vi "subSwitches.vi"(1 "AxisId":i32=1, 2 "Index":i32=1) -> ()   [LabVIEW 2020]
panel:
  out "LimMaxSt":bool caption="S-MAX"
  out "LimMinSt":bool caption="S-MIN"
  in  "MaxPos":i32
  in  "MinPos":i32
  in  "LimMax":bool caption="S-MAX"
  in  "LimMin":bool caption="S-MIN"
  in  "REF4":bool caption="MAXSTP"
  in  "REF3":bool caption="MAXDEC"
  in  "REF2":bool caption="MINDEC"
  in  "REF1":bool caption="MINSTP"
  in  "RH4":bool caption="High"
  in  "RL4":bool caption="Low"
  in  "RH3":bool caption="High"
  in  "RL3":bool caption="Low"
  in  "RH2":bool caption="High"
  in  "RL2":bool caption="Low"
  in  "RH1":bool caption="High"
  in  "RL1":bool caption="Low"
  in  "MaxDec":bool caption="MAXDEC"
  in  "MinDec":bool caption="MINDEC"
  in  "MaxStop":bool caption="MAXSTOP"
  in  "MinStop":bool caption="MINSTOP"
  out "MaxDecSt":bool caption="MAXDEC"
  out "MinDecSt":bool caption="MINDEC"
  in  "Save":bool
  in  "H4":bool caption="High"
  in  "L4":bool caption="Low"
  in  "H3":bool caption="High"
  in  "L3":bool caption="Low"
  in  "H2":bool caption="High"
  in  "L2":bool caption="Low"
  in  "H1":bool caption="High"
  in  "L1":bool caption="Low"
  out "MaxStopSt":bool caption="MAXSTP"
  out "MinStopSt":bool caption="MINSTP"
  out "Hyst":i32 caption="Limit switch hysteresis"
  in  "Close":bool
  # "Axis"
  # "State (activated?)"
  # "Limit switches (mask + polarity)"
  # "Ref switch (mask + polarity)"
  # "Software limits"
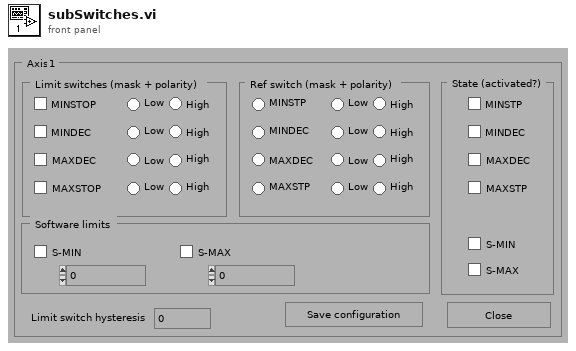
[diagram p1: front panel]
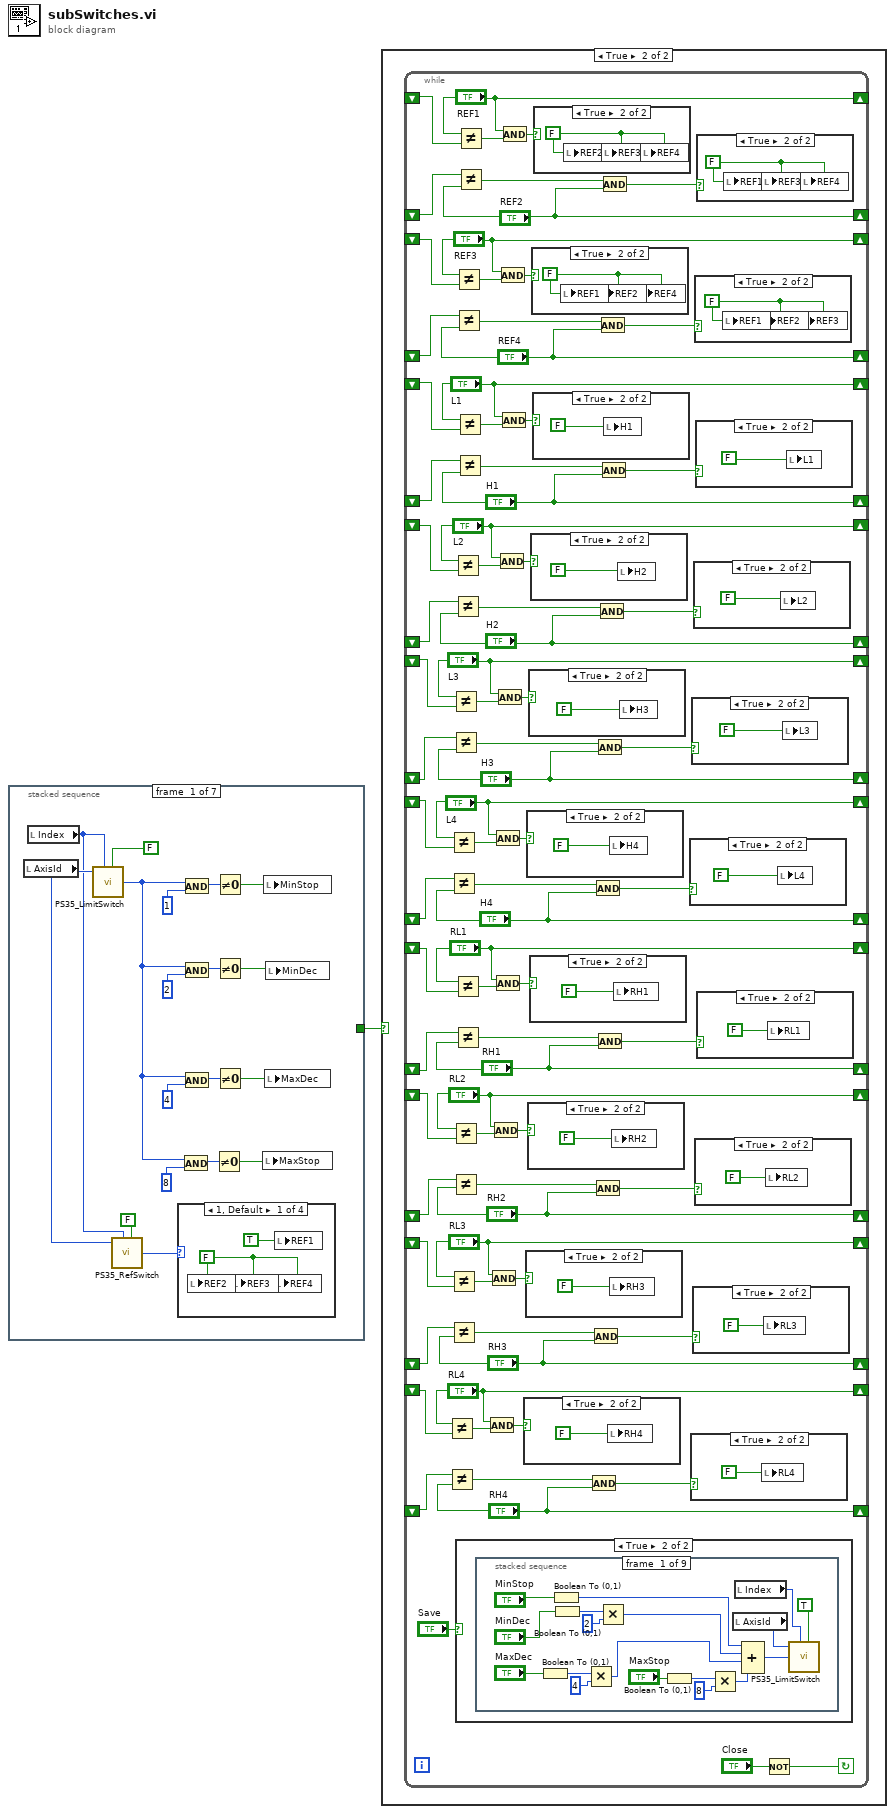
[diagram p0: block diagram]
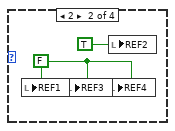
[diagram p2: hidden frame]
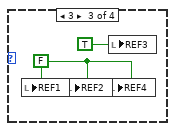
[diagram p3: hidden frame]
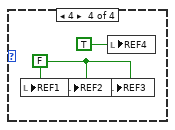
[diagram p4: hidden frame]
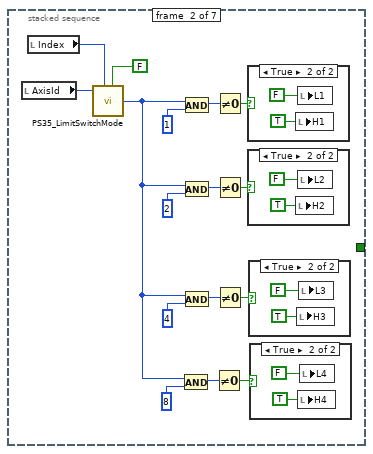
[diagram p5: hidden frame]
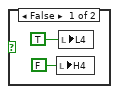
[diagram p6: hidden frame]
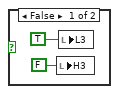
[diagram p7: hidden frame]
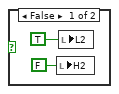
[diagram p8: hidden frame]
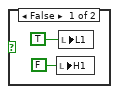
[diagram p9: hidden frame]
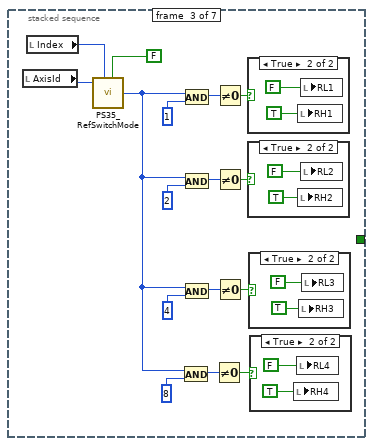
[diagram p10: hidden frame]
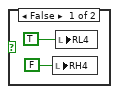
[diagram p11: hidden frame]
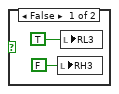
[diagram p12: hidden frame]
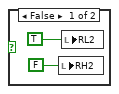
[diagram p13: hidden frame]
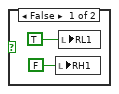
[diagram p14: hidden frame]
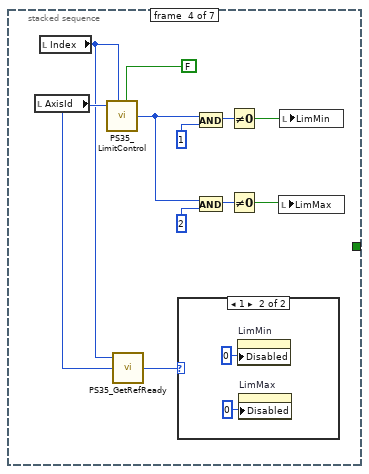
[diagram p15: hidden frame]
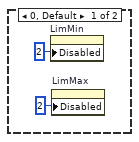
[diagram p16: hidden frame]
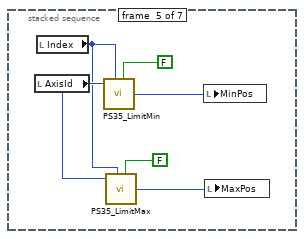
[diagram p17: hidden frame]
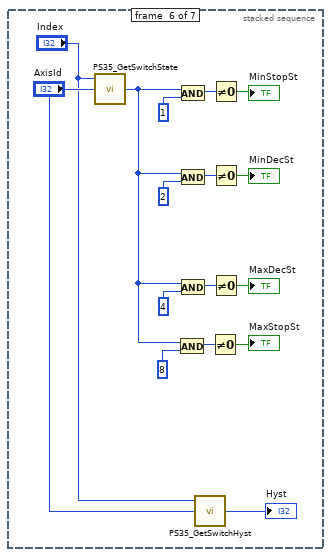
[diagram p18: hidden frame]
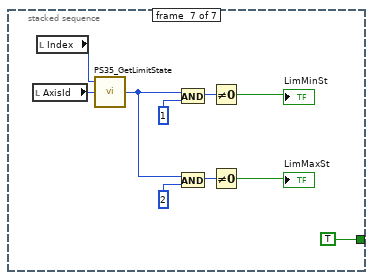
[diagram p19: hidden frame]
diagram:
  n1 = stacked-sequence {
    tunnel: [_ _ _ _ _ _ TRUE] -> w1
    frame #0 {
      n2 = local read "AxisId"() -> (w3:i32)
      n3 = local read "Index"() -> (w2:i32)
      n4 = call "PS35_LimitSwitch.vi"("Axis number"=w3, "Control unit ID"=w2, "function"=FALSE ("WriteRead")) -> ("Value-Out"=w10:i32)  [unwired: 5 in, 1 out]
      n5 = call "PS35_RefSwitch.vi"("Axis number"=w3, "Control unit ID"=w2, "function"=FALSE ("WriteRead")) -> ("Value-Out"=w4:i32)  [unwired: 5 in, 1 out]
      n6 = case shown="1, Default" w4 {
        frame 1, Default {
          w20 = FALSE
          n7 = local write "REF2"(w20) -> ()
          n8 = local write "REF3"(w20) -> ()
          n9 = local write "REF4"(w20) -> ()
          n10 = local write "REF1"(TRUE) -> ()
        }
        frame 2 {
          w22 = FALSE
          n11 = local write "REF1"(w22) -> ()
          n12 = local write "REF3"(w22) -> ()
          n13 = local write "REF4"(w22) -> ()
          n14 = local write "REF2"(TRUE) -> ()
        }
        frame 3 {
          w24 = FALSE
          n15 = local write "REF1"(w24) -> ()
          n16 = local write "REF2"(w24) -> ()
          n17 = local write "REF4"(w24) -> ()
          n18 = local write "REF3"(TRUE) -> ()
        }
        frame 4 {
          w26 = FALSE
          n19 = local write "REF1"(w26) -> ()
          n20 = local write "REF2"(w26) -> ()
          n21 = local write "REF3"(w26) -> ()
          n22 = local write "REF4"(TRUE) -> ()
        }
      }
      n23 = And(x=w10, y=8) -> (x .and. y?=w11:i32)
      n24 = And(x=w10, y=1) -> (x .and. y?=w18:i32)
      n25 = And(x=w10, y=2) -> (x .and. y?=w15:i32)
      n26 = And(x=w10, y=4) -> (x .and. y?=w14:i32)
      n27 = Not Equal To 0?(x=w11) -> (x != 0?=w6:bool)
      n28 = Not Equal To 0?(x=w18) -> (x != 0?=w9:bool)
      n29 = Not Equal To 0?(x=w15) -> (x != 0?=w8:bool)
      n30 = Not Equal To 0?(x=w14) -> (x != 0?=w7:bool)
      n31 = local write "MaxStop"(w6) -> ()
      n32 = local write "MinStop"(w9) -> ()
      n33 = local write "MaxDec"(w7) -> ()
      n34 = local write "MinDec"(w8) -> ()
    }
    frame #1 {
      n35 = local read "AxisId"() -> (w29:i32)
      n36 = local read "Index"() -> (w28:i32)
      n37 = call "PS35_LimitSwitchMode.vi"("Axis number"=w29, "Control unit ID"=w28, "function"=FALSE ("WriteRead")) -> ("Value-Out"=w33:i32)  [unwired: 5 in, 1 out]
      n38 = And(x=w33, y=8) -> (x .and. y?=w34:i32)
      n39 = And(x=w33, y=1) -> (x .and. y?=w41:i32)
      n40 = And(x=w33, y=2) -> (x .and. y?=w38:i32)
      n41 = And(x=w33, y=4) -> (x .and. y?=w37:i32)
      n42 = Not Equal To 0?(x=w34) -> (x != 0?=w31:bool)
      n43 = Not Equal To 0?(x=w41) -> (x != 0?=w42:bool)
      n44 = Not Equal To 0?(x=w38) -> (x != 0?=w32:bool)
      n45 = Not Equal To 0?(x=w37) -> (x != 0?=w30:bool)
      n46 = case shown="True" w42 {
        frame False {
          n47 = local write "H1"(FALSE ("PLS12")) -> ()
          n48 = local write "L1"(TRUE ("PLS11")) -> ()
        }
        frame True {
          n49 = local write "H1"(TRUE ("PLS12")) -> ()
          n50 = local write "L1"(FALSE ("PLS11")) -> ()
        }
      }
      n51 = case shown="True" w32 {
        frame False {
          n52 = local write "H2"(FALSE ("PLS12")) -> ()
          n53 = local write "L2"(TRUE ("PLS11")) -> ()
        }
        frame True {
          n54 = local write "H2"(TRUE ("PLS12")) -> ()
          n55 = local write "L2"(FALSE ("PLS11")) -> ()
        }
      }
      n56 = case shown="True" w30 {
        frame False {
          n57 = local write "H3"(FALSE ("PLS12")) -> ()
          n58 = local write "L3"(TRUE ("PLS11")) -> ()
        }
        frame True {
          n59 = local write "H3"(TRUE ("PLS12")) -> ()
          n60 = local write "L3"(FALSE ("PLS11")) -> ()
        }
      }
      n61 = case shown="True" w31 {
        frame False {
          n62 = local write "H4"(FALSE ("PLS12")) -> ()
          n63 = local write "L4"(TRUE ("PLS11")) -> ()
        }
        frame True {
          n64 = local write "H4"(TRUE ("PLS12")) -> ()
          n65 = local write "L4"(FALSE ("PLS11")) -> ()
        }
      }
    }
    frame #2 {
      n66 = local read "AxisId"() -> (w61:i32)
      n67 = local read "Index"() -> (w60:i32)
      n68 = call "PS35_RefSwitchMode.vi"("Axis number"=w61, "Control unit ID"=w60, "function"=FALSE ("WriteRead")) -> ("Value-Out"=w65:i32)  [unwired: 5 in, 1 out]
      n69 = And(x=w65, y=8) -> (x .and. y?=w66:i32)
      n70 = And(x=w65, y=1) -> (x .and. y?=w73:i32)
      n71 = And(x=w65, y=2) -> (x .and. y?=w70:i32)
      n72 = And(x=w65, y=4) -> (x .and. y?=w69:i32)
      n73 = Not Equal To 0?(x=w66) -> (x != 0?=w62:bool)
      n74 = Not Equal To 0?(x=w73) -> (x != 0?=w74:bool)
      n75 = Not Equal To 0?(x=w70) -> (x != 0?=w64:bool)
      n76 = Not Equal To 0?(x=w69) -> (x != 0?=w63:bool)
      n77 = case shown="True" w74 {
        frame False {
          n78 = local write "RH1"(FALSE ("PLS12")) -> ()
          n79 = local write "RL1"(TRUE ("PLS11")) -> ()
        }
        frame True {
          n80 = local write "RH1"(TRUE ("PLS12")) -> ()
          n81 = local write "RL1"(FALSE ("PLS11")) -> ()
        }
      }
      n82 = case shown="True" w64 {
        frame False {
          n83 = local write "RH2"(FALSE ("PLS12")) -> ()
          n84 = local write "RL2"(TRUE ("PLS11")) -> ()
        }
        frame True {
          n85 = local write "RH2"(TRUE ("PLS12")) -> ()
          n86 = local write "RL2"(FALSE ("PLS11")) -> ()
        }
      }
      n87 = case shown="True" w63 {
        frame False {
          n88 = local write "RH3"(FALSE ("PLS12")) -> ()
          n89 = local write "RL3"(TRUE ("PLS11")) -> ()
        }
        frame True {
          n90 = local write "RH3"(TRUE ("PLS12")) -> ()
          n91 = local write "RL3"(FALSE ("PLS11")) -> ()
        }
      }
      n92 = case shown="True" w62 {
        frame False {
          n93 = local write "RH4"(FALSE ("PLS12")) -> ()
          n94 = local write "RL4"(TRUE ("PLS11")) -> ()
        }
        frame True {
          n95 = local write "RH4"(TRUE ("PLS12")) -> ()
          n96 = local write "RL4"(FALSE ("PLS11")) -> ()
        }
      }
    }
    frame #3 {
      n97 = local read "AxisId"() -> (w93:i32)
      n98 = local read "Index"() -> (w92:i32)
      n99 = call "PS35_LimitControl.vi"("Axis number"=w93, "Control unit ID"=w92, "function"=FALSE ("WriteRead")) -> ("Value-Out"=w97:i32)  [unwired: 5 in, 1 out]
      n100 = call "PS35_GetRefReady.vi"("Axis number"=w93, "Control unit ID"=w92) -> ("State"=w94:i32)  [unwired: 2 in, 1 out]
      n101 = case shown="1" w94 {
        frame 0, Default {
          n102 = property on="LimMin" class="Bool (strict)"("Disabled"=u8 2) -> ()  [unwired: 2 in, 2 out]
          n103 = property on="LimMax" class="Bool (strict)"("Disabled"=u8 2) -> ()  [unwired: 2 in, 2 out]
        }
        frame 1 {
          n104 = property on="LimMin" class="Bool (strict)"("Disabled"=u8 0) -> ()  [unwired: 2 in, 2 out]
          n105 = property on="LimMax" class="Bool (strict)"("Disabled"=u8 0) -> ()  [unwired: 2 in, 2 out]
        }
      }
      n106 = And(x=w97, y=1) -> (x .and. y?=w101:i32)
      n107 = And(x=w97, y=2) -> (x .and. y?=w98:i32)
      n108 = Not Equal To 0?(x=w101) -> (x != 0?=w96:bool)
      n109 = Not Equal To 0?(x=w98) -> (x != 0?=w95:bool)
      n110 = local write "LimMax"(w95) -> ()
      n111 = local write "LimMin"(w96) -> ()
    }
    frame #4 {
      n112 = local read "AxisId"() -> (w108:i32)
      n113 = local read "Index"() -> (w107:i32)
      n114 = call "PS35_LimitMin.vi"("Axis number"=w108, "Control unit ID"=w107, "function"=FALSE ("WriteRead")) -> ("Value-Out"=w110:i32)  [unwired: 5 in, 1 out]
      n115 = call "PS35_LimitMax.vi"("Axis number"=w108, "Control unit ID"=w107, "function"=FALSE ("WriteRead")) -> ("Value-Out"=w111:i32)  [unwired: 5 in, 1 out]
      n116 = local write "MinPos"(w110) -> ()
      n117 = local write "MaxPos"(w111) -> ()
    }
    frame #5 {
      n118 = call "PS35_GetSwitchState.vi"("Axis number"="AxisId", "Control unit ID"="Index") -> ("Switch state"=w119:i32)  [unwired: 2 in, 1 out]
      n119 = And(x=w119, y=8) -> (x .and. y?=w120:i32)
      n120 = And(x=w119, y=1) -> (x .and. y?=w127:i32)
      n121 = And(x=w119, y=2) -> (x .and. y?=w124:i32)
      n122 = And(x=w119, y=4) -> (x .and. y?=w123:i32)
      n123 = call "PS35_GetSwitchHyst.vi"("Axis number"="AxisId", "Control unit ID"="Index") -> ("Value"=→"Hyst":i32)  [unwired: 2 in, 1 out]
      n124 = Not Equal To 0?(x=w120) -> (x != 0?=→"MaxStopSt":bool)
      n125 = Not Equal To 0?(x=w127) -> (x != 0?=→"MinStopSt":bool)
      n126 = Not Equal To 0?(x=w124) -> (x != 0?=→"MinDecSt":bool)
      n127 = Not Equal To 0?(x=w123) -> (x != 0?=→"MaxDecSt":bool)
    }
    frame #6 {
      n128 = local read "AxisId"() -> (w133:i32)
      n129 = local read "Index"() -> (w129:i32)
      n130 = call "PS35_GetLimitState.vi"("Axis number"=w133, "Control unit ID"=w129) -> ("Limit state"=w132:i32)  [unwired: 2 in, 1 out]
      n131 = And(x=w132, y=1) -> (x .and. y?=w137:i32)
      n132 = And(x=w132, y=2) -> (x .and. y?=w134:i32)
      n133 = Not Equal To 0?(x=w137) -> (x != 0?=→"LimMinSt":bool)
      n134 = Not Equal To 0?(x=w134) -> (x != 0?=→"LimMaxSt":bool)
    }
  }
  n135 = case shown="True" w1 {
    frame False {
      (unwired) FALSE ("End")
    }
    frame True {
      n136 = while {
        shift-left: _ -> [w159]
        shift-right: ["REF4"] -> _
        shift-left: _ -> [w164]
        shift-right: ["REF3"] -> _
        shift-left: _ -> [w158]
        shift-right: ["REF2"] -> _
        shift-left: _ -> [w153]
        shift-right: ["REF1"] -> _
        shift-left: _ -> [w166]
        shift-right: ["RL4"] -> _
        shift-left: _ -> [w165]
        shift-right: ["RH4"] -> _
        shift-left: _ -> [w168]
        shift-right: ["RL3"] -> _
        shift-left: _ -> [w167]
        shift-right: ["RH3"] -> _
        shift-left: _ -> [w170]
        shift-right: ["RL2"] -> _
        shift-left: _ -> [w169]
        shift-right: ["RH2"] -> _
        shift-left: _ -> [w172]
        shift-right: ["RL1"] -> _
        shift-left: _ -> [w171]
        shift-right: ["RH1"] -> _
        shift-left: _ -> [w200]
        shift-right: ["H4"] -> _
        shift-left: _ -> [w205]
        shift-right: ["L4"] -> _
        shift-left: _ -> [w147]
        shift-right: ["H3"] -> _
        shift-left: _ -> [w195]
        shift-right: ["L3"] -> _
        shift-left: _ -> [w211]
        shift-right: ["H2"] -> _
        shift-left: _ -> [w186]
        shift-right: ["L2"] -> _
        shift-left: _ -> [w212]
        shift-right: ["H1"] -> _
        shift-left: _ -> [w219]
        shift-right: ["L1"] -> _
        stop <- w220 continue-if-true
        n137 = Not Equal?(x="RL4", y=w166) -> (x != y?=w180:bool)
        n138 = Not Equal?(x=w165, y="RH4") -> (x != y?=w177:bool)
        n139 = Not Equal?(x="L4", y=w205) -> (x != y?=w204:bool)
        n140 = Not Equal?(x=w200, y="H4") -> (x != y?=w202:bool)
        n141 = Not Equal?(x="RL3", y=w168) -> (x != y?=w173:bool)
        n142 = Not Equal?(x=w167, y="RH3") -> (x != y?=w176:bool)
        n143 = Not Equal?(x="L3", y=w195) -> (x != y?=w196:bool)
        n144 = Not Equal?(x=w147, y="H3") -> (x != y?=w198:bool)
        n145 = Not Equal?(x="RL2", y=w170) -> (x != y?=w181:bool)
        n146 = Not Equal?(x=w169, y="RH2") -> (x != y?=w184:bool)
        n147 = Not Equal?(x="L2", y=w186) -> (x != y?=w207:bool)
        n148 = Not Equal?(x=w211, y="H2") -> (x != y?=w209:bool)
        n149 = Not Equal?(x="RL1", y=w172) -> (x != y?=w190:bool)
        n150 = Not Equal?(x=w171, y="RH1") -> (x != y?=w187:bool)
        n151 = Not Equal?(x="REF3", y=w164) -> (x != y?=w163:bool)
        n152 = Not Equal?(x=w159, y="REF4") -> (x != y?=w161:bool)
        n153 = Not Equal?(x="L1", y=w219) -> (x != y?=w218:bool)
        n154 = Not Equal?(x=w212, y="H1") -> (x != y?=w215:bool)
        n155 = Not Equal?(x="REF1", y=w153) -> (x != y?=w154:bool)
        n156 = Not Equal?(x=w158, y="REF2") -> (x != y?=w156:bool)
        n157 = case shown="True" "Save" {
          frame False {
            n158 = Wait (ms)(milliseconds to wait=u32 200) -> ()  [unwired: 1 out]
          }
          frame True {
            n159 = stacked-sequence {
              frame #0 {
                n160 = Boolean To (0,1)(Boolean="MaxDec") -> (0, 1=w244:i16)
                n161 = Boolean To (0,1)(Boolean="MinStop") -> (0, 1=w250:i16)
                n162 = Boolean To (0,1)(Boolean="MinDec") -> (0, 1=w247:i16)
                n163 = Multiply(x=w244, y=i16 4) -> (x*y=w239:i16)
                n164 = Multiply(x=w247, y=i16 2) -> (x*y=w240:i16)
                n165 = Boolean To (0,1)(Boolean="MaxStop") -> (0, 1=w243:i16)
                n166 = Multiply(x=w243, y=i16 8) -> (x*y=w237:i16)
                n167 = local read "AxisId"() -> (w236:i32)
                n168 = local read "Index"() -> (w235:i32)
                n169 = Compound Arithmetic op=ADD(w250, w240, w239, w237) -> (w249:i16)
                n170 = call "PS35_LimitSwitch.vi"("Axis number"=w236, "Control unit ID"=w235, "Value-In"=w249, "function"=TRUE ("WriteRead")) -> ()  [unwired: 4 in, 2 out]
              }
              frame #1 {
                n171 = local read "H1"() -> (w258:bool)
                n172 = local read "H2"() -> (w255:bool)
                n173 = local read "H3"() -> (w257:bool)
                n174 = Boolean To (0,1)(Boolean=w257) -> (0, 1=w264:i16)
                n175 = Boolean To (0,1)(Boolean=w258) -> (0, 1=w269:i16)
                n176 = Boolean To (0,1)(Boolean=w255) -> (0, 1=w267:i16)
                n177 = Multiply(x=w264, y=i16 4) -> (x*y=w260:i16)
                n178 = Multiply(x=w267, y=i16 2) -> (x*y=w261:i16)
                n179 = local read "H4"() -> (w256:bool)
                n180 = Boolean To (0,1)(Boolean=w256) -> (0, 1=w263:i16)
                n181 = Multiply(x=w263, y=i16 8) -> (x*y=w259:i16)
                n182 = local read "AxisId"() -> (w254:i32)
                n183 = local read "Index"() -> (w253:i32)
                n184 = Compound Arithmetic op=ADD(w269, w261, w260, w259) -> (w268:i16)
                n185 = call "PS35_LimitSwitchMode.vi"("Axis number"=w254, "Control unit ID"=w253, "Value-In"=w268, "function"=TRUE ("WriteRead")) -> ()  [unwired: 4 in, 2 out]
              }
              frame #2 {
                n186 = local read "RH1"() -> (w276:bool)
                n187 = local read "RH2"() -> (w273:bool)
                n188 = local read "RH3"() -> (w275:bool)
                n189 = Boolean To (0,1)(Boolean=w275) -> (0, 1=w282:i16)
                n190 = Boolean To (0,1)(Boolean=w276) -> (0, 1=w287:i16)
                n191 = Boolean To (0,1)(Boolean=w273) -> (0, 1=w285:i16)
                n192 = Multiply(x=w282, y=i16 4) -> (x*y=w278:i16)
                n193 = Multiply(x=w285, y=i16 2) -> (x*y=w279:i16)
                n194 = local read "RH4"() -> (w274:bool)
                n195 = Boolean To (0,1)(Boolean=w274) -> (0, 1=w281:i16)
                n196 = Multiply(x=w281, y=i16 8) -> (x*y=w277:i16)
                n197 = local read "AxisId"() -> (w272:i32)
                n198 = local read "Index"() -> (w271:i32)
                n199 = Compound Arithmetic op=ADD(w287, w279, w278, w277) -> (w286:i16)
                n200 = call "PS35_RefSwitchMode.vi"("Axis number"=w272, "Control unit ID"=w271, "Value-In"=w286, "function"=TRUE ("WriteRead")) -> ()  [unwired: 4 in, 2 out]
              }
              frame #3 {
                n201 = local read "REF1"() -> (w294:bool)
                n202 = local read "REF2"() -> (w291:bool)
                n203 = local read "REF3"() -> (w293:bool)
                n204 = Boolean To (0,1)(Boolean=w293) -> (0, 1=w300:i16)
                n205 = Boolean To (0,1)(Boolean=w294) -> (0, 1=w305:i16)
                n206 = Boolean To (0,1)(Boolean=w291) -> (0, 1=w303:i16)
                n207 = Multiply(x=w300, y=i16 3) -> (x*y=w296:i16)
                n208 = Multiply(x=w303, y=i16 2) -> (x*y=w297:i16)
                n209 = local read "REF4"() -> (w292:bool)
                n210 = Boolean To (0,1)(Boolean=w292) -> (0, 1=w299:i16)
                n211 = Multiply(x=w299, y=i16 4) -> (x*y=w295:i16)
                n212 = local read "AxisId"() -> (w290:i32)
                n213 = local read "Index"() -> (w289:i32)
                n214 = Compound Arithmetic op=ADD(w305, w297, w296, w295) -> (w304:i16)
                n215 = call "PS35_RefSwitch.vi"("Axis number"=w290, "Control unit ID"=w289, "Value-In"=w304, "function"=TRUE ("WriteRead")) -> ()  [unwired: 4 in, 2 out]
              }
              frame #4 {
                n216 = Boolean To (0,1)(Boolean="LimMin") -> (0, 1=w315:i16)
                n217 = Boolean To (0,1)(Boolean="LimMax") -> (0, 1=w313:i16)
                n218 = Multiply(x=w313, y=i16 2) -> (x*y=w311:i16)
                n219 = local read "Index"() -> (w307:i32)
                n220 = local read "AxisId"() -> (w310:i32)
                n221 = Compound Arithmetic op=ADD(w315, w311) -> (w314:i16)
                n222 = call "PS35_LimitControl.vi"("Axis number"=w310, "Control unit ID"=w307, "Value-In"=w314, "function"=TRUE ("WriteRead")) -> ()  [unwired: 4 in, 2 out]
              }
              frame #5 {
                n223 = local read "AxisId"() -> (w319:i32)
                n224 = local read "Index"() -> (w317:i32)
                n225 = call "PS35_LimitMin.vi"("Axis number"=w319, "Control unit ID"=w317, "Value-In"="MinPos", "function"=TRUE ("WriteRead")) -> ()  [unwired: 4 in, 2 out]
              }
              frame #6 {
                n226 = local read "AxisId"() -> (w323:i32)
                n227 = local read "Index"() -> (w321:i32)
                n228 = call "PS35_LimitMax.vi"("Axis number"=w323, "Control unit ID"=w321, "Value-In"="MaxPos", "function"=TRUE ("WriteRead")) -> ()  [unwired: 4 in, 2 out]
              }
              frame #7 {
                n229 = local read "AxisId"() -> (w326:i32)
                n230 = local read "Index"() -> (w325:i32)
                n231 = call "PS35_GetSwitchState.vi"("Axis number"=w326, "Control unit ID"=w325) -> ("Switch state"=w330:i32)  [unwired: 2 in, 1 out]
                n232 = And(x=w330, y=1) -> (x .and. y?=w338:i32)
                n233 = And(x=w330, y=2) -> (x .and. y?=w336:i32)
                n234 = Not Equal To 0?(x=w338) -> (x != 0?=w337:bool)
                n235 = And(x=w330, y=4) -> (x .and. y?=w333:i32)
                n236 = Not Equal To 0?(x=w336) -> (x != 0?=w329:bool)
                n237 = And(x=w330, y=8) -> (x .and. y?=w332:i32)
                n238 = Not Equal To 0?(x=w333) -> (x != 0?=w328:bool)
                n239 = Not Equal To 0?(x=w332) -> (x != 0?=w327:bool)
                n240 = local write "MinStopSt"(w337) -> ()
                n241 = local write "MinDecSt"(w329) -> ()
                n242 = local write "MaxDecSt"(w328) -> ()
                n243 = local write "MaxStopSt"(w327) -> ()
              }
              frame #8 {
                n244 = local read "AxisId"() -> (w342:i32)
                n245 = local read "Index"() -> (w340:i32)
                n246 = call "PS35_GetLimitState.vi"("Axis number"=w342, "Control unit ID"=w340) -> ("Limit state"=w341:i32)  [unwired: 2 in, 1 out]
                n247 = And(x=w341, y=1) -> (x .and. y?=w347:i32)
                n248 = And(x=w341, y=2) -> (x .and. y?=w345:i32)
                n249 = Not Equal To 0?(x=w347) -> (x != 0?=w346:bool)
                n250 = Not Equal To 0?(x=w345) -> (x != 0?=w343:bool)
                n251 = local write "LimMinSt"(w346) -> ()
                n252 = local write "LimMaxSt"(w343) -> ()
              }
            }
          }
        }
        n253 = And(x="RL4", y=w180) -> (x .and. y?=w179:bool)
        n254 = And(x="RL3", y=w173) -> (x .and. y?=w174:bool)
        n255 = And(x="RL2", y=w181) -> (x .and. y?=w182:bool)
        n256 = And(x="L4", y=w204) -> (x .and. y?=w203:bool)
        n257 = And(x="RL1", y=w190) -> (x .and. y?=w189:bool)
        n258 = And(x="L3", y=w196) -> (x .and. y?=w197:bool)
        n259 = And(x="L2", y=w207) -> (x .and. y?=w208:bool)
        n260 = And(x="REF3", y=w163) -> (x .and. y?=w162:bool)
        n261 = And(x="L1", y=w218) -> (x .and. y?=w216:bool)
        n262 = And(x="REF1", y=w154) -> (x .and. y?=w155:bool)
        n263 = case shown="True" w179 {
          frame False {
          }
          frame True {
            n264 = local write "RH4"(FALSE) -> ()
          }
        }
        n265 = case shown="True" w174 {
          frame False {
          }
          frame True {
            n266 = local write "RH3"(FALSE) -> ()
          }
        }
        n267 = case shown="True" w203 {
          frame False {
          }
          frame True {
            n268 = local write "H4"(FALSE) -> ()
          }
        }
        n269 = case shown="True" w182 {
          frame False {
          }
          frame True {
            n270 = local write "RH2"(FALSE) -> ()
          }
        }
        n271 = case shown="True" w197 {
          frame False {
          }
          frame True {
            n272 = local write "H3"(FALSE) -> ()
          }
        }
        n273 = case shown="True" w189 {
          frame False {
          }
          frame True {
            n274 = local write "RH1"(FALSE) -> ()
          }
        }
        n275 = case shown="True" w208 {
          frame False {
          }
          frame True {
            n276 = local write "H2"(FALSE) -> ()
          }
        }
        n277 = case shown="True" w162 {
          frame False {
          }
          frame True {
            w225 = FALSE
            n278 = local write "REF1"(w225) -> ()
            n279 = local write "REF2"(w225) -> ()
            n280 = local write "REF4"(w225) -> ()
          }
        }
        n281 = case shown="True" w216 {
          frame False {
          }
          frame True {
            n282 = local write "H1"(FALSE) -> ()
          }
        }
        n283 = case shown="True" w155 {
          frame False {
          }
          frame True {
            w222 = FALSE
            n284 = local write "REF2"(w222) -> ()
            n285 = local write "REF3"(w222) -> ()
            n286 = local write "REF4"(w222) -> ()
          }
        }
        n287 = And(x=w177, y="RH4") -> (x .and. y?=w178:bool)
        n288 = And(x=w176, y="RH3") -> (x .and. y?=w175:bool)
        n289 = And(x=w202, y="H4") -> (x .and. y?=w201:bool)
        n290 = And(x=w184, y="RH2") -> (x .and. y?=w183:bool)
        n291 = And(x=w198, y="H3") -> (x .and. y?=w199:bool)
        n292 = And(x=w187, y="RH1") -> (x .and. y?=w188:bool)
        n293 = And(x=w209, y="H2") -> (x .and. y?=w210:bool)
        n294 = And(x=w161, y="REF4") -> (x .and. y?=w160:bool)
        n295 = And(x=w215, y="H1") -> (x .and. y?=w213:bool)
        n296 = And(x=w156, y="REF2") -> (x .and. y?=w157:bool)
        n297 = case shown="True" w201 {
          frame False {
          }
          frame True {
            n298 = local write "L4"(FALSE) -> ()
          }
        }
        n299 = case shown="True" w178 {
          frame False {
          }
          frame True {
            n300 = local write "RL4"(FALSE) -> ()
          }
        }
        n301 = case shown="True" w199 {
          frame False {
          }
          frame True {
            n302 = local write "L3"(FALSE) -> ()
          }
        }
        n303 = case shown="True" w175 {
          frame False {
          }
          frame True {
            n304 = local write "RL3"(FALSE) -> ()
          }
        }
        n305 = case shown="True" w210 {
          frame False {
          }
          frame True {
            n306 = local write "L2"(FALSE) -> ()
          }
        }
        n307 = case shown="True" w160 {
          frame False {
          }
          frame True {
            w224 = FALSE
            n308 = local write "REF1"(w224) -> ()
            n309 = local write "REF2"(w224) -> ()
            n310 = local write "REF3"(w224) -> ()
          }
        }
        n311 = case shown="True" w183 {
          frame False {
          }
          frame True {
            n312 = local write "RL2"(FALSE) -> ()
          }
        }
        n313 = case shown="True" w213 {
          frame False {
          }
          frame True {
            n314 = local write "L1"(FALSE) -> ()
          }
        }
        n315 = case shown="True" w157 {
          frame False {
          }
          frame True {
            w223 = FALSE
            n316 = local write "REF1"(w223) -> ()
            n317 = local write "REF3"(w223) -> ()
            n318 = local write "REF4"(w223) -> ()
          }
        }
        n319 = case shown="True" w188 {
          frame False {
          }
          frame True {
            n320 = local write "RL1"(FALSE) -> ()
          }
        }
        n321 = Not(x="Close") -> (.not. x?=w220:bool)
      }
    }
  }
